vi "Build Frame Script Core.vi"(8 "error in (no error)":errorcluster, 10 "Config Strings":string[](array[string]), 11 "BML Pattern Creater in":refnum<class "BML Pattern Creater.lvclass">) -> (0 "error out":errorcluster, 2 "Pattern Script":string, 3 "BML Pattern Creater out":refnum<class "BML Pattern Creater.lvclass">)   [LabVIEW 2018, in "BML Pattern Creater.lvlib" / "BML Pattern Creater.lvclass"]
uses:
  BML Pattern Creater.lvclass
  C:/P4 Workspace/PC Client/Solutions/5g_eap/trunk/1.0/HiSi5GmmWave/Pattern_Gen_Tool/Interfaces/Protocol Interface.lvlibp/Interfaces/Protocol Interface/Protocol Interface.lvclass
  Special Frame.ctl
  Interfaces/Protocol Interface.lvlibp/Interfaces/Protocol Interface/Read Wait(ms).vi
  Interfaces/Protocol Interface.lvlibp/Interfaces/Protocol Interface/Read Period(ms).vi
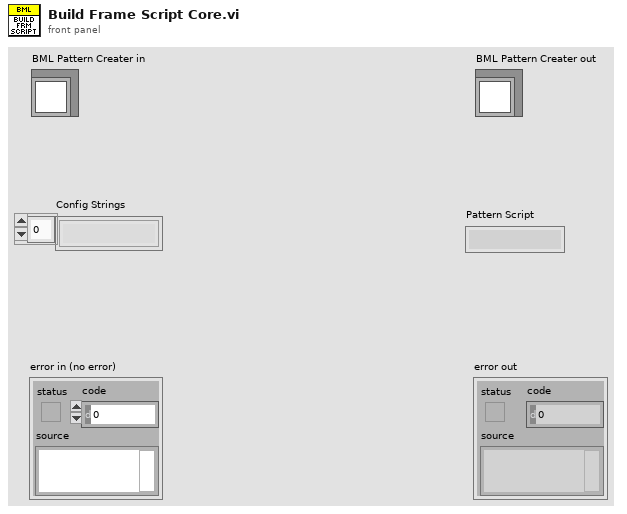
[diagram p1: front panel]
types:
  T1 = typedef "BML Pattern Creater.lvlib/BML Pattern Creater.lvclass/Special Frame.ctl" = enum16{"Sync Header", "BML Header", "SW Trig", "SetID State", "Exit SetID State", "SW Reset", "Wait"}
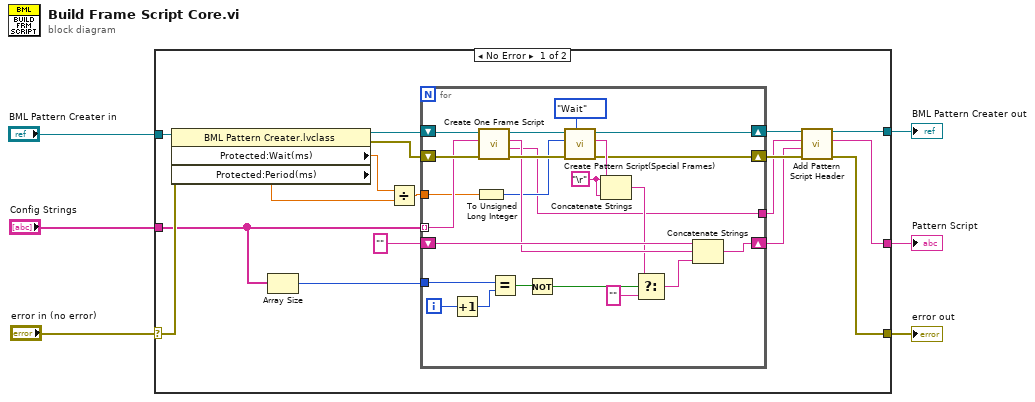
[diagram p0: block diagram]
diagram:
  n1 = case shown="No Error" "error in (no error)" {
    selector: "error in (no error)" -> [w22 w48]
    tunnel: "BML Pattern Creater in" -> [w23 w49]
    tunnel: "Config Strings" -> [w16 _]
    tunnel: [w13 w49] -> w2
    tunnel: [w8 w48] -> w3
    tunnel: [w9 _] -> w1
    frame No Error {
      n2 = property class="BML Pattern Creater.lvclass"(reference=w23, error in=w22) -> (reference out=w21:refnum<class "BML Pattern Creater.lvclass">, error out=w18:errorcluster, "Protected:Wait(ms)"=w7:dbl, "Protected:Period(ms)"=w20:dbl)
      n3 = Array Size(array=w16) -> (size(s)=w15:i32)
      n4 = Divide(x=w7, y=w20) -> (x/y=w19:dbl)
      n5 = for {
        tunnel: w16 -> [w45] mode=indexing
        shift-right: [w27] -> w12
        shift-left: w18 -> [w46]
        tunnel: w19 -> [w26]
        shift-right: [w41] -> w14
        shift-left: w21 -> [w47]
        shift-right: [w40] -> w10
        shift-left: "" -> [w36]
        tunnel: w15 -> [w39]
        tunnel: [w24] -> w11
        i -> [w38]
        w29 = "\r"
        n6 = Increment(x=w38) -> (x+1=w37:i32)
        n7 = To Unsigned Long Integer(number=w26) -> (unsigned 32bit integer=w25:u32)
        n8 = call-dynamic "Create One Frame Script.vi"("error in (no error)"=w46, "Config String"=w45, "BML Pattern Creater in"=w47) -> ("error out"=w42:errorcluster, "Pattern Name out"=w24:string, "Script out"=w33:string, "BML Pattern Creater out"=w43:refnum<class "BML Pattern Creater.lvclass">)  [unwired: 5 in]
        n9 = Equal?(x=w39, y=w37) -> (x = y?=w35:bool)
        n10 = Not(x=w35) -> (.not. x?=w34:bool)
        n11 = call "Create Pattern Script(Special Frames).vi"("Special Frame Type"=Special_Frame."Wait", "error in (no error)"=w42, "Num of Timeset"=w25, "BML Pattern Creater in"=w43) -> ("error out"=w27:errorcluster, "string out"=w32:string, "BML Pattern Creater out"=w41:refnum<class "BML Pattern Creater.lvclass">)  [unwired: 5 in]
        n12 = Concatenate Strings(w29, w32, w29) -> (w31:string)
        n13 = Select(t=w31, s=w34, f="") -> (s? t:f=w30:string)
        n14 = Concatenate Strings(w36, w33, w30) -> (w40:string)
      }
      n15 = call "Add Pattern Script Header.vi"("error in (no error)"=w12, "Pattern Script Frame in"=w10, "Pattern Name"=w11, "BML Pattern Creater"=w14) -> ("error out"=w8:errorcluster, "Pattern Script All out"=w9:string, "BML Pattern Creater"=w13:refnum<class "BML Pattern Creater.lvclass">)  [unwired: 5 in]
    }
    frame Error {
    }
  }
  "error out" <- w3
  "BML Pattern Creater out" <- w2
  "Pattern Script" <- w1
